vi "Copy Scripting API to Installed Location.vi"(5 "Files Generated by Build":path[](array[path]), 6 "Top Level/Always Included VIs":path[](array[path]), 7 "Destination Path":path, 8 "error in (no error)":errorcluster, 9 "Target Name":string, 10 "Build Specification Name":string, 11 "Project Path":path) -> (0 "error out":errorcluster)   [LabVIEW 2020]
doc: "This VI is called after each run of a build specification. The VI will copy the generated LLB (Engine or System Explorer) into the VeriStand Custom Device folder (...\\Documents\\National Instruments\\NI VeriStand 2013...)."
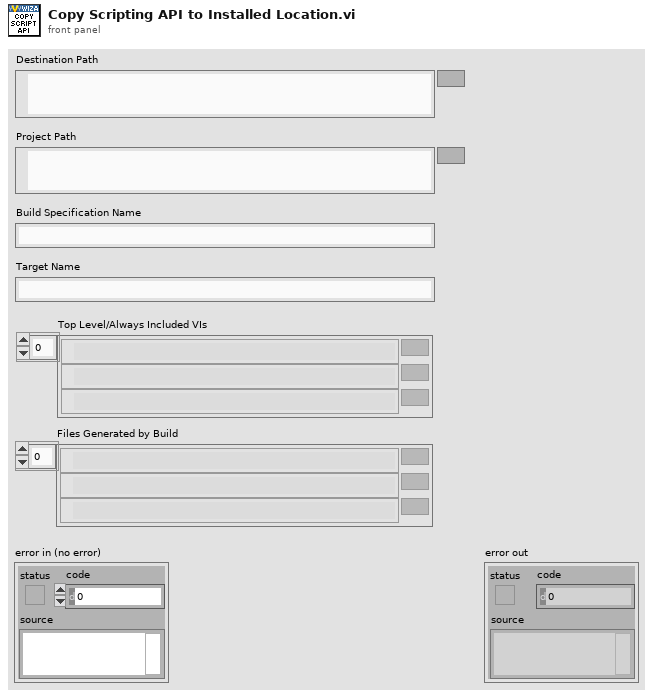
[diagram p1: front panel]
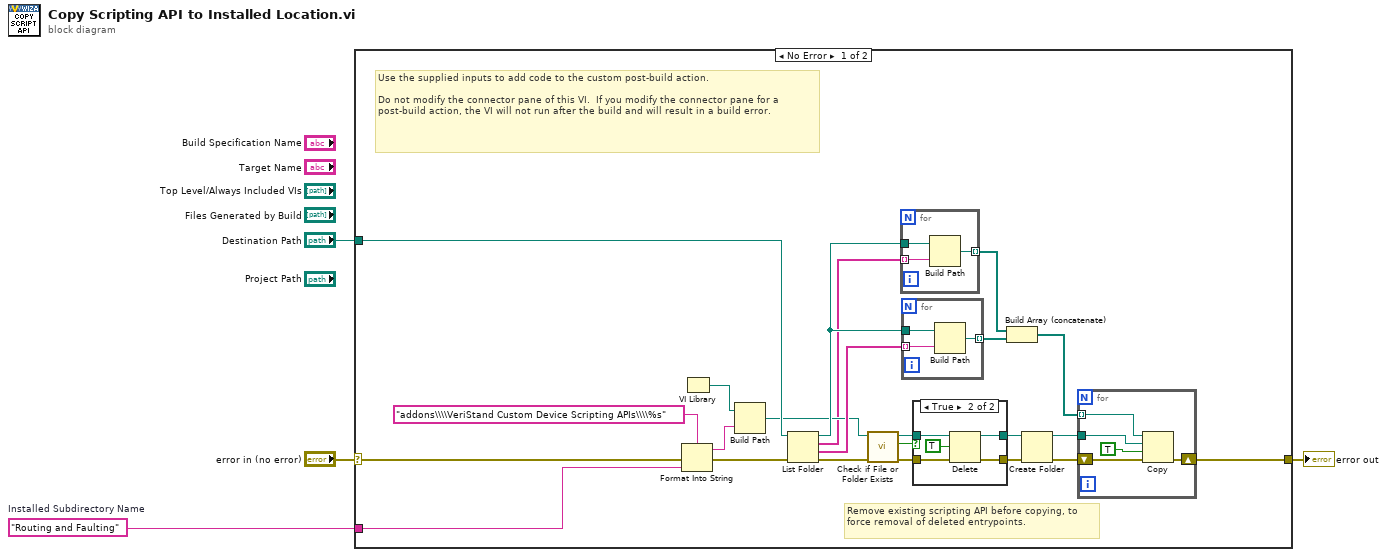
[diagram p0: block diagram]
diagram:
  w3 = "Routing and Faulting"  # Installed Subdirectory Name
  n1 = case shown="No Error" "error in (no error)" {
    selector: "error in (no error)" -> [w27 w46]
    tunnel: [w25 w46] -> w2
    tunnel: w3 -> [w26 _]
    tunnel: "Destination Path" -> [w24 _]
    frame No Error {
      # "Remove existing scripting API before copying, to force removal of deleted entrypoints."
      # "Use the supplied inputs to add code to the custom post-build action.\n\nDo not modify the connector pane of this VI.  If you modify the connector pane for a post-build action, the VI will not run after the build and will result in a build error."
      n2 = Format Into String(format string="addons\\\\VeriStand Custom Device Scripting APIs\\\\%s" ("name or relative path"), error in=w27, w26) -> (resulting string=w17:string, error out=w14:errorcluster)  [unwired: 1 in]
      n3 = VI Library() -> (path=w12:path)
      n4 = Build Path(base path=w12, name or relative path=w17) -> (appended path=w15:path)
      n5 = List Folder(path=w24, error in=w14) -> (path out=w20:path, filenames=w13:string[], folder names=w21:string[], error out=w18:errorcluster)  [unwired: 2 in]
      n6 = call <vilib>:"Check if File or Folder Exists.vi"("error in (no error)"=w18, "path"=w15) -> ("error out"=w7:errorcluster, "file or folder exists?"=w9:bool, "dup path"=w8:path)  [unwired: 7 in]
      n7 = for {
        tunnel: w13 -> [w39] mode=indexing
        tunnel: w20 -> [w40]
        tunnel: [w38] -> w23 mode=indexing
        n8 = Build Path(base path=w40, name or relative path=w39) -> (appended path=w38:path)
      }
      n9 = for {
        tunnel: w21 -> [w36] mode=indexing
        tunnel: w20 -> [w37]
        tunnel: [w35] -> w19 mode=indexing
        n10 = Build Path(base path=w37, name or relative path=w36) -> (appended path=w35:path)
      }
      n11 = case shown="True" w9 {
        tunnel: w8 -> [w29 w34]
        tunnel: w7 -> [w28 w33]
        tunnel: [w29 w32] -> w11
        tunnel: [w28 w31] -> w10
        frame False {
        }
        frame True {
          n12 = Delete(path (use dialog)=w34, entire hierarchy (F)=TRUE, error in=w33) -> (deleted path=w32:path, error out=w31:errorcluster)  [unwired: 2 in, 1 out]
        }
      }
      n13 = Build Array (concatenate)(w23, w19) -> (w22:path[])
      n14 = Create Folder(path (use dialog)=w11, error in=w10) -> (created path=w5:path, error out=w6:errorcluster)  [unwired: 1 in, 1 out]
      n15 = for {
        tunnel: w22 -> [w42] mode=indexing
        shift-right: [w43] -> w25
        shift-left: w6 -> [w44]
        tunnel: w5 -> [w41]
        n16 = Copy(8:w44, 9:TRUE ("overwrite (F)"), 10:w41, 11:w42) -> (0:w43:errorcluster)  [unwired: 1 in, 2 out]
      }
    }
    frame Error {
    }
  }
  "error out" <- w2
